vi "Write to Motor State Reference.vi"(8 "error in (no error)":errorcluster, 9 "state mode":T1 items=["undefined", "angle", "velocity"], 10 "value":dbl, 11 "motor state ref in":refnum<data-value>) -> (0 "error out":errorcluster, 1 "failed?":bool, 3 "motor state ref out":refnum<data-value>)   [LabVIEW 2017, in "NI_Robotics_Motor Communication Ref.lvclass"]
uses:
  <vilib>/robotics/Actuation/Motor Communication Ref/NI_Robotics_Motor Communication Ref.lvclass
  <vilib>/robotics/Actuation/Motor Communication/Motor State Value.ctl
  <vilib>/robotics/Actuation/Motor Communication/Motor State Mode.ctl
  <vilib>/robotics/Actuation/Motor Communication/NI_Robotics_Motor Communication.lvclass
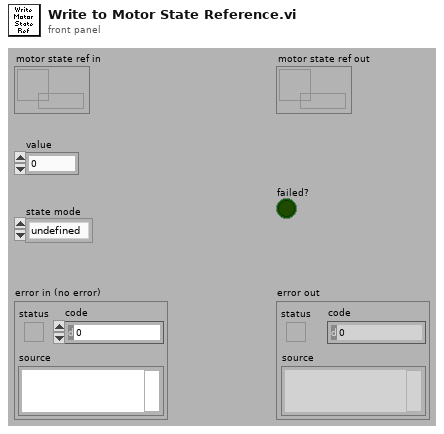
[diagram p1: front panel]
types:
  T1 = typedef "NI_Robotics_Motor Communication.lvclass/Motor State Mode.ctl" = u16
  T2 = typedef "NI_Robotics_Motor Communication.lvclass/Motor State Value.ctl" = cluster{"angle":dbl, "velocity":dbl, "state mode":T1}
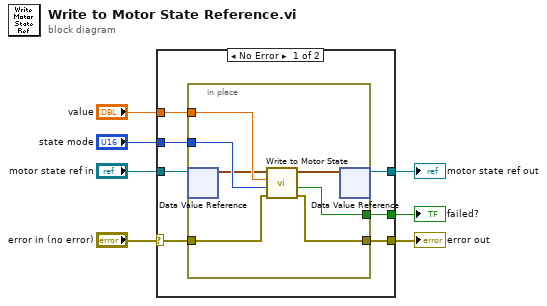
[diagram p0: block diagram]
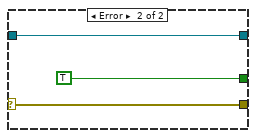
[diagram p2: hidden frame]
diagram:
  n1 = case shown="No Error" "error in (no error)" {
    selector: "error in (no error)" -> [w9 w23]
    tunnel: "motor state ref in" -> [w14 w24]
    tunnel: [w13 w24] -> w5
    tunnel: [w8 w23] -> w4
    tunnel: "state mode" -> [w12 _]
    tunnel: "value" -> [w11 _]
    tunnel: [w10 TRUE] -> w1
    frame No Error {
      n2 = in-place {
        in-place-border: w12 -> [w20]
        in-place-border: w11 -> [w21]
        in-place-border: [w18] -> w10
        in-place-border: w9 -> [w16]
        in-place-border: [w15] -> w8
        n3 = in-place-dvr #1(w14) -> (w19:T2)  [unwired: 1 out]
        n4 = call <vilib>:"Write to Motor State.vi"("error in (no error)"=w16, "state mode"=w20, "value"=w21, "motor state in"=w19) -> ("error out"=w15:errorcluster, "failed?"=w18:bool, "motor state out"=w17:T2)  [unwired: 5 in]
        n5 = in-place-dvr #1(w17) -> (w13:refnum<data-value>)  [unwired: 1 out]
      }
    }
    frame Error {
    }
  }
  "motor state ref out" <- w5
  "error out" <- w4
  "failed?" <- w1
